vi "Transport.vi"(4 "Queue of Async Elements":refnum<queue>, 6 "Actor Ref":refnum<vi>, 7 "Actor in":refnum<class "Actor.lvclass">, 9 "Attributes":refnum<class "Attributes.lvclass">, 10 "Refs":refnum<class "Refs.lvclass">) -> (0 "Error out":errorcluster, 5 "Actor out":refnum<class "Actor.lvclass">)   [LabVIEW 2025, in "jettl.lvlib" / "Queue Transport.lvlib"]
uses:
  Queue Transport.lvlib
  Actor/Actor.lvclass
  Attributes/Attributes.lvclass
  Refs/Refs.lvclass
  Async Elements.ctl
  Msg Output/Msg Output.lvclass
  jettl.lvlib
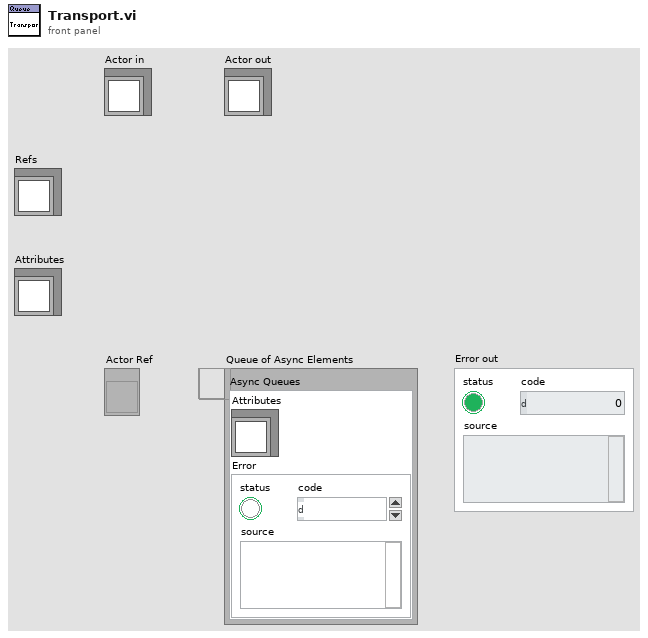
[diagram p1: front panel]
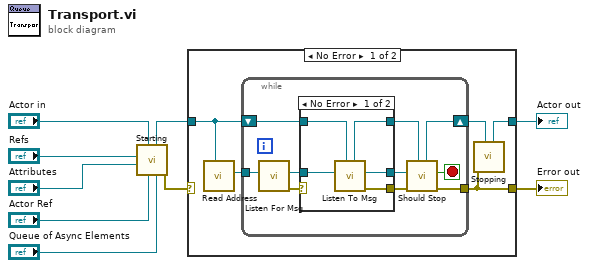
[diagram p0: block diagram]
diagram:
  n1 = call "Starting.vi"("Queue of Async Elements"="Queue of Async Elements", "Actor Ref"="Actor Ref", "Actor in"="Actor in", "Attributes"="Attributes", "Refs"="Refs") -> ("Error out"=w5:errorcluster, "Actor out"=w7:refnum<class "Actor.lvclass">)  [unwired: 5 in]
  n2 = case shown="No Error" w5 {
    selector: w5 -> [_ w33]
    tunnel: [w12 w32] -> w8
    tunnel: [w14 w33] -> w9
    tunnel: w7 -> [w10 w32]
    frame No Error {
      n3 = call "Read Address.vi"("Actor"=w10) -> ("Address"=w11:refnum<data-value>)  [unwired: 10 in]
      n4 = while {
        shift-right: [w22] -> w13
        shift-left: w10 -> [w20]
        tunnel: [w23] -> w14
        tunnel: w11 -> [w18]
        stop <- w21 stop-if-true
        n5 = call "Listen For Msg.vi"("Address"=w18) -> ("Error out"=w16:errorcluster, "Msg"=w17:refnum<class "Msg.lvclass">)  [unwired: 9 in]
        n6 = case shown="No Error" w16 {
          selector: w16 -> [_ w30]
          tunnel: [w26 w30] -> w24
          tunnel: w20 -> [w29 w31]
          tunnel: [w27 w31] -> w19
          tunnel: w17 -> [w28 _]
          tunnel: [w25 _] -> w15
          frame No Error {
            n7 = call "Listen To Msg.vi"("Actor in"=w29, "Msg"=w28) -> ("Error out"=w26:errorcluster, "Msg Output"=w25:refnum<class "Msg Output.lvclass">, "Actor out"=w27:refnum<class "Actor.lvclass">)  [unwired: 7 in]
          }
          frame Error {
          }
        }
        n8 = call "Should Stop.vi"("Actor in"=w19, "Error in"=w24, "Msg Output"=w15) -> ("Error out"=w23:errorcluster, "Stop"=w21:bool, "Actor out"=w22:refnum<class "Actor.lvclass">)  [unwired: 6 in]
      }
      n9 = call "Stopping.vi"("Actor in"=w13, "Error in"=w14) -> ("Actor out"=w12:refnum<class "Actor.lvclass">)  [unwired: 9 in]
    }
    frame Error {
    }
  }
  "Error out" <- w9
  "Actor out" <- w8
